vi "lv9_daqusb6251.vi"() -> ()   [LabVIEW 2021]
panel:
  out "teste":dynamicdata(graph)=[{"t0"=timestamp(3730382840.471822 s since 1904-01-01), "dt"=1.0, "Y"=[-0.00023800805463109788]}]
  out "Dinamômetro":string
  out "error out":errorcluster
  in  "VISA resource name":refnum<visa-resource-name>
  out "Final time [s]":dbl
  out "Iteration":i32
  out "Waveform Chart 2":dynamicdata(graph)=[{"t0"=timestamp(3730382840.471822 s since 1904-01-01), "dt"=1.0, "Y"=[-0.00023800805463109788]}]
  in  "Device name":tag="Dev1"
  in  "Number of samples \nto read":i32=1000
  in  "Acquisition rate [Hz]":dbl=100.0
  out "Waveform Chart":dynamicdata(graph)=[{"t0"=timestamp(3730382840.471822 s since 1904-01-01), "dt"=1.0, "Y"=[-0.23734714614383248]}]
  in  "Stop":bool
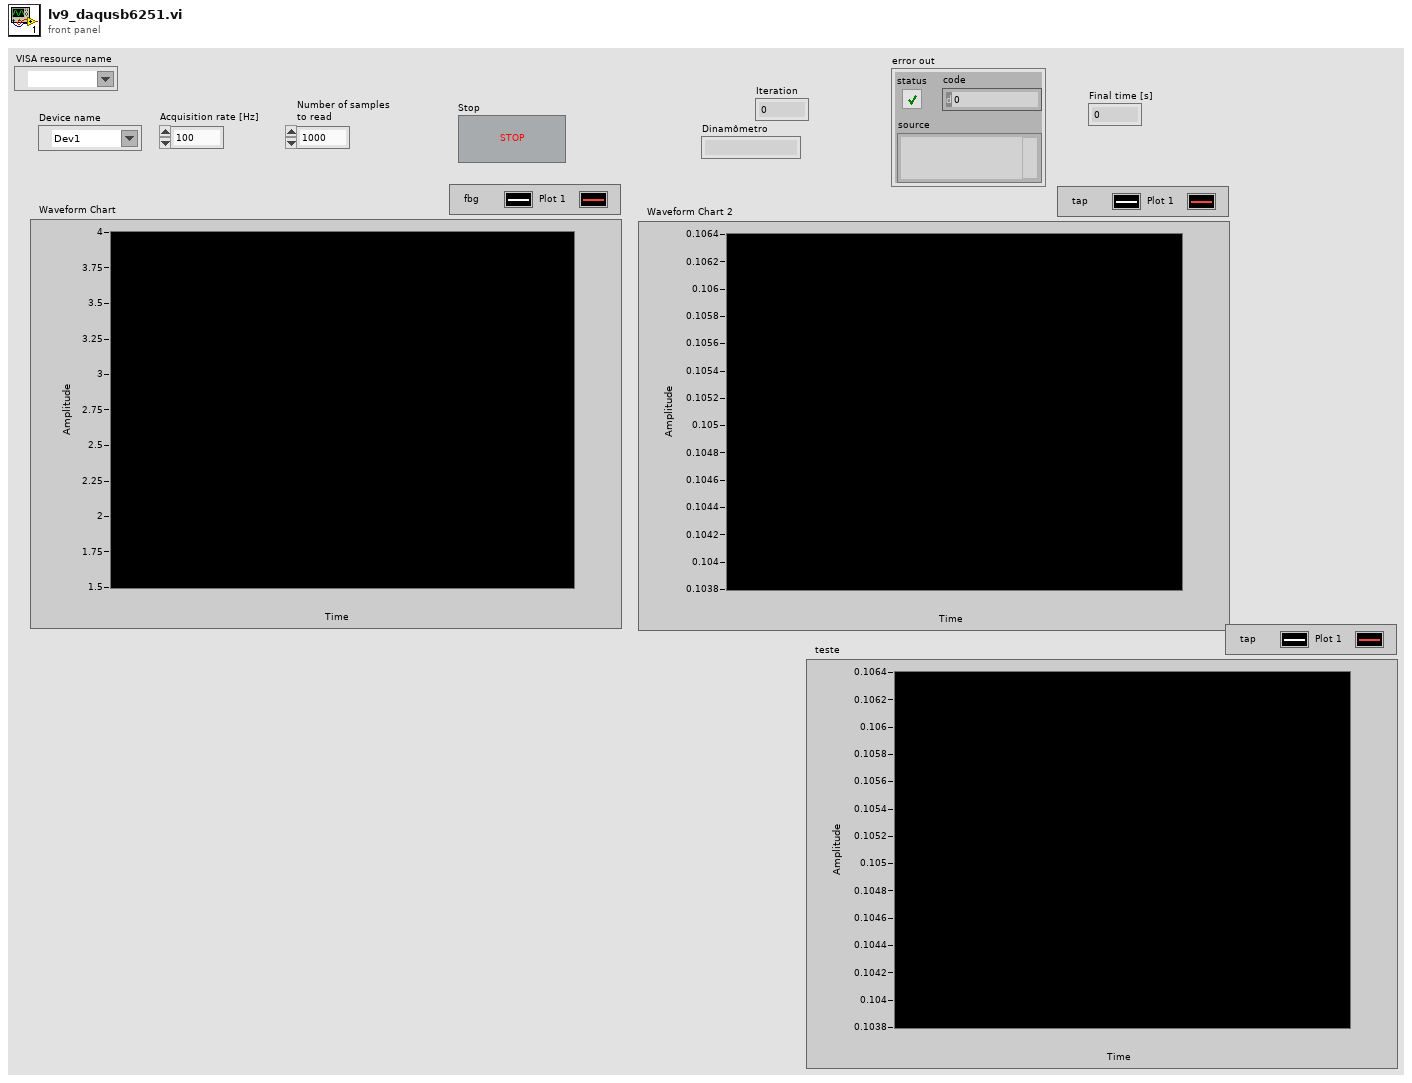
[diagram p1: front panel]
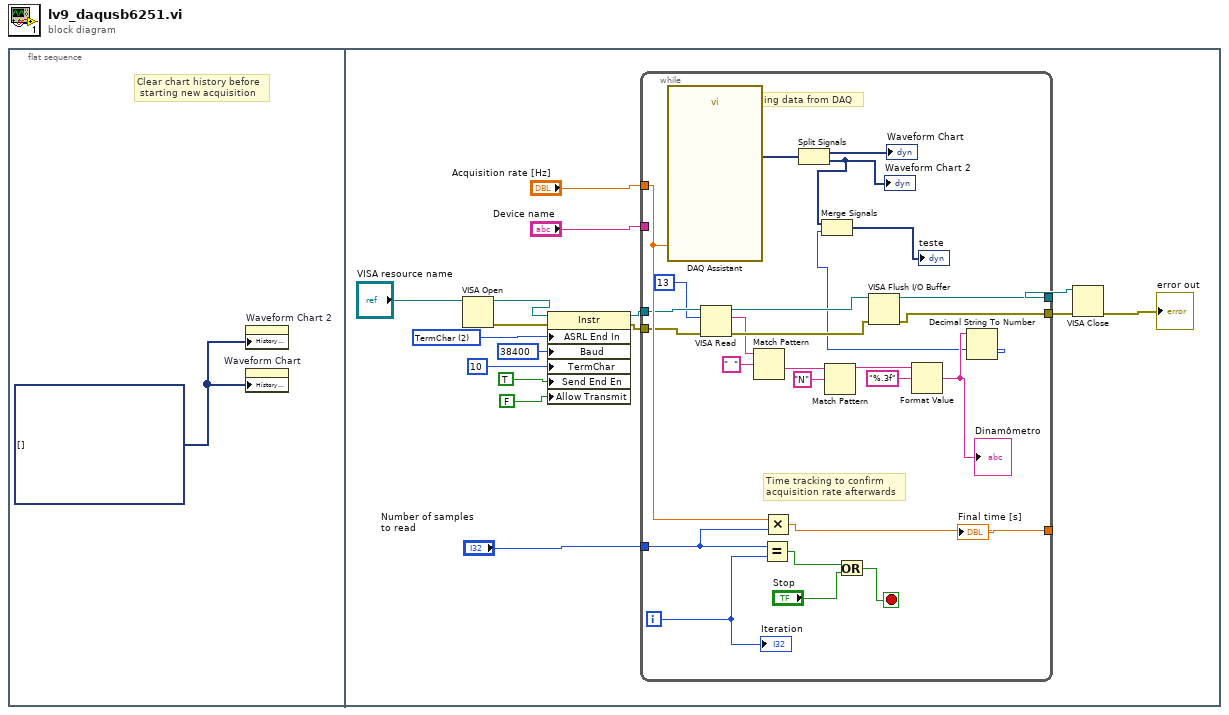
[diagram p0: block diagram]
diagram:
  n1 = flat-sequence {
    frame #0 {
      w1 = dynamicdata[] [] ("History Data")
      # "Clear chart history before\n starting new acquisition"
      n2 = property on="Waveform Chart 2" class="WFChart (strict)"("History Data"=w1) -> ()  [unwired: 2 in, 2 out]
      n3 = property on="Waveform Chart" class="WFChart (strict)"("History Data"=w1) -> ()  [unwired: 2 in, 2 out]
    }
    frame #1 {
      w4 = u16 2 items=["None", "Last Bit", "TermChar"] ("Serial Settings:End Mode for Reads")
      n4 = VISA Open(VISA resource name="VISA resource name") -> (VISA resource name=w7:refnum<visa-resource-name>, error out=w8:errorcluster)  [unwired: 4 in]
      n5 = property class="Instr"(reference=w7, error in=w8, "ASRL End In"=w4, "Baud"=u32 38400 ("Serial Settings:Baud Rate"), "TermChar"=u8 10 ("Message Based Settings:Termination Character"), "Send End En"=TRUE, "Allow Transmit"=FALSE) -> (reference out=w10:refnum<visa-resource-name>, error out=w9:errorcluster)
      n6 = while {
        tunnel: "Device name" -> [_]
        tunnel: "Number of samples \nto read" -> [w38]
        tunnel: [w37] -> w17
        tunnel: "Acquisition rate [Hz]" -> [w36]
        tunnel: [w34] -> w14
        tunnel: [w32] -> w12
        tunnel: w10 -> [w31]
        tunnel: w9 -> [w30]
        i -> [w40]
        stop <- w41 stop-if-true
        # "Reading data from DAQ"
        # "Time tracking to confirm\nacquisition rate afterwards"
        n7 = call "DAQ Assistant"("rate"=w36) -> ("data"=w43:dynamicdata)  [unwired: 15 in, 3 out]
        n8 = VISA Read(VISA resource name=w31, byte count=u32 13, error in (no error)=w30) -> (VISA resource name out=w35:refnum<visa-resource-name>, read buffer=w28:string, error out=w33:errorcluster)  [unwired: 1 out]
        n9 = Match Pattern(string=w28, regular expression="  ") -> (after substring=w26:string)  [unwired: 1 in, 3 out]
        n10 = Equal?(x=w38, y=w40) -> (x = y?=w39:bool)
        n11 = Multiply(x=w36, y=w38) -> (x*y=w37:dbl)
        n12 = Split Signals(w43) -> (→"Waveform Chart":dynamicdata, w21:dynamicdata)  [unwired: 2 in]
        "Waveform Chart 2" <- w21
        n13 = Match Pattern(string=w26, regular expression="N") -> (before substring=w24:string)  [unwired: 1 in, 3 out]
        n14 = Or(x=w39, y="Stop") -> (x .or. y?=w41:bool)
        n15 = VISA Flush I/O Buffer(VISA resource name=w35, error in (no error)=w33) -> (VISA resource name out=w34:refnum<visa-resource-name>, error out=w32:errorcluster)  [unwired: 1 in]
        n16 = Format Value(string ("")=w24, format string="%.3f") -> (output string=w22:string)  [unwired: 1 in]
        "Dinamômetro" <- w22
        n17 = Decimal String To Number(string=w22) -> (number=w20:i32)  [unwired: 2 in, 1 out]
        n18 = Merge Signals(w21, w20) -> (→"teste":dynamicdata)
        "Iteration" <- w40
      }
      "Final time [s]" <- w17
      n19 = VISA Close(VISA resource name=w14, error in (no error)=w12) -> (error out=→"error out":errorcluster)
    }
  }
